vi "AnalyzeLineSpeed.vi"(1 "Line Length [mm]":dbl format="%#_13g", 2 "Line Speeds [mm/s]":T2) -> (0 "Output":T1)   [LabVIEW 2017]
panel:
  out "Motion Time [s]":dbl
  out "Vy [mm/s]":dbl
  out "Vx [mm/s]":dbl
  out "V [mm/s]":dbl
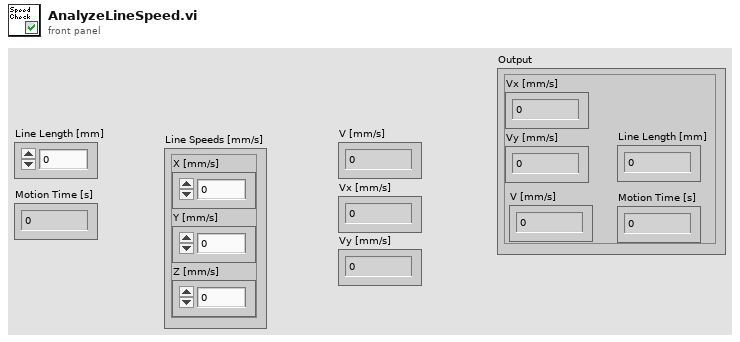
[diagram p1: front panel]
types:
  T1 = cluster{"Vx [mm/s]":dbl, "Vy [mm/s]":dbl, "Numeric Control":dbl, "Numeric Control":dbl, "Line Length [mm]":dbl}
  T2 = cluster{"X [mm/s]":dbl, "Y [mm/s]":dbl, "Z [mm/s]":dbl}
  T3 = cluster{"X [mm/s]":dbl, "Y [mm/s]":dbl, dbl, dbl, "Line Length [mm]":dbl}
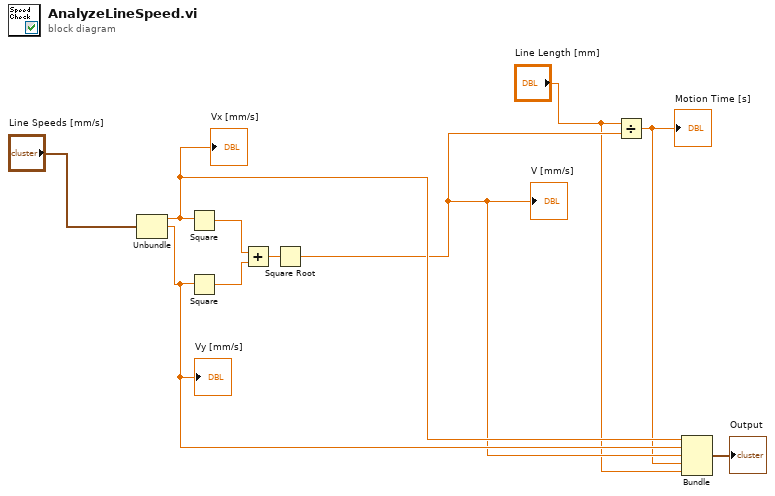
[diagram p0: block diagram]
diagram:
  n1 = Unbundle("Line Speeds [mm/s]") -> ("X [mm/s]"=w6:dbl, "Y [mm/s]"=w5:dbl)  [unwired: 1 out]
  "Vx [mm/s]" <- w6
  "Vy [mm/s]" <- w5
  n2 = Square(x=w6) -> (x^2=w9:dbl)
  n3 = Square(x=w5) -> (x^2=w8:dbl)
  n4 = Add(x=w9, y=w8) -> (x+y=w7:dbl)
  n5 = Square Root(x=w7) -> (sqrt(x)=w4:dbl)
  "V [mm/s]" <- w4
  n6 = Divide(x="Line Length [mm]", y=w4) -> (x/y=w3:dbl)
  "Motion Time [s]" <- w3
  n7 = Bundle("X [mm/s]"=w6, "Y [mm/s]"=w5, w4, w3, "Line Length [mm]"="Line Length [mm]") -> (→"Output":T3)  [unwired: 1 in]
